vi "get_image.vi"(9 "Input\nparameters":T2={"Frame rate (ms)"=2000, "Worm Strain"="N2", "Time t"=0, "State"=enum."Image acquisition", "Acquisition time"=0.0, "Maximum # of images"=100000, "#TTL"=0, "time of third ttl "=100000, "ImSub Value"=0, "Time of last TTL"=0, "# Rows"=2, "# Columns"=2, "number of adjacentTTL"=0, "Sleep Deprivation status"="", "Sleep Detection"=FALSE, "Time of first sleep detection"=0, "# Sleep detections"=0, "Time max # adjacent TTL"=-10000, "Image t-1"=[], "Image t"=[]} {"# Columns" items=["1"=1, "2"=2, "3"=3, "4"=4]; "# Rows" items=["1"=1, "2"=2, "3"=3, "4"=4]}, 10 "?":bool) -> (1 "Output\nparameters":T2={"Frame rate (ms)"=2000, "Worm Strain"="N2", "Time t"=0, "State"=enum."Image acquisition", "Acquisition time"=0.0, "Maximum # of images"=100000, "#TTL"=0, "time of third ttl "=100000, "ImSub Value"=0, "Time of last TTL"=0, "# Rows"=2, "# Columns"=2, "number of adjacentTTL"=0, "Sleep Deprivation status"="", "Sleep Detection"=FALSE, "Time of first sleep detection"=0, "# Sleep detections"=0, "Time max # adjacent TTL"=-10000, "Image t-1"=[], "Image t"=[]} {"# Columns" items=["1"=1, "2"=2, "3"=3, "4"=4]; "# Rows" items=["1"=1, "2"=2, "3"=3, "4"=4]}, 5 "Intensity Graph":u16[][](graph))   [LabVIEW 2011]
uses:
  state.ctl
panel:
  out "?":i32
  out "?":i32
  # "General settings"
  # "Select number of animals"
  # "Row"
  # "Column"
  # "General settings"
  # "Select number of animals"
  # "Row"
  # "Column"
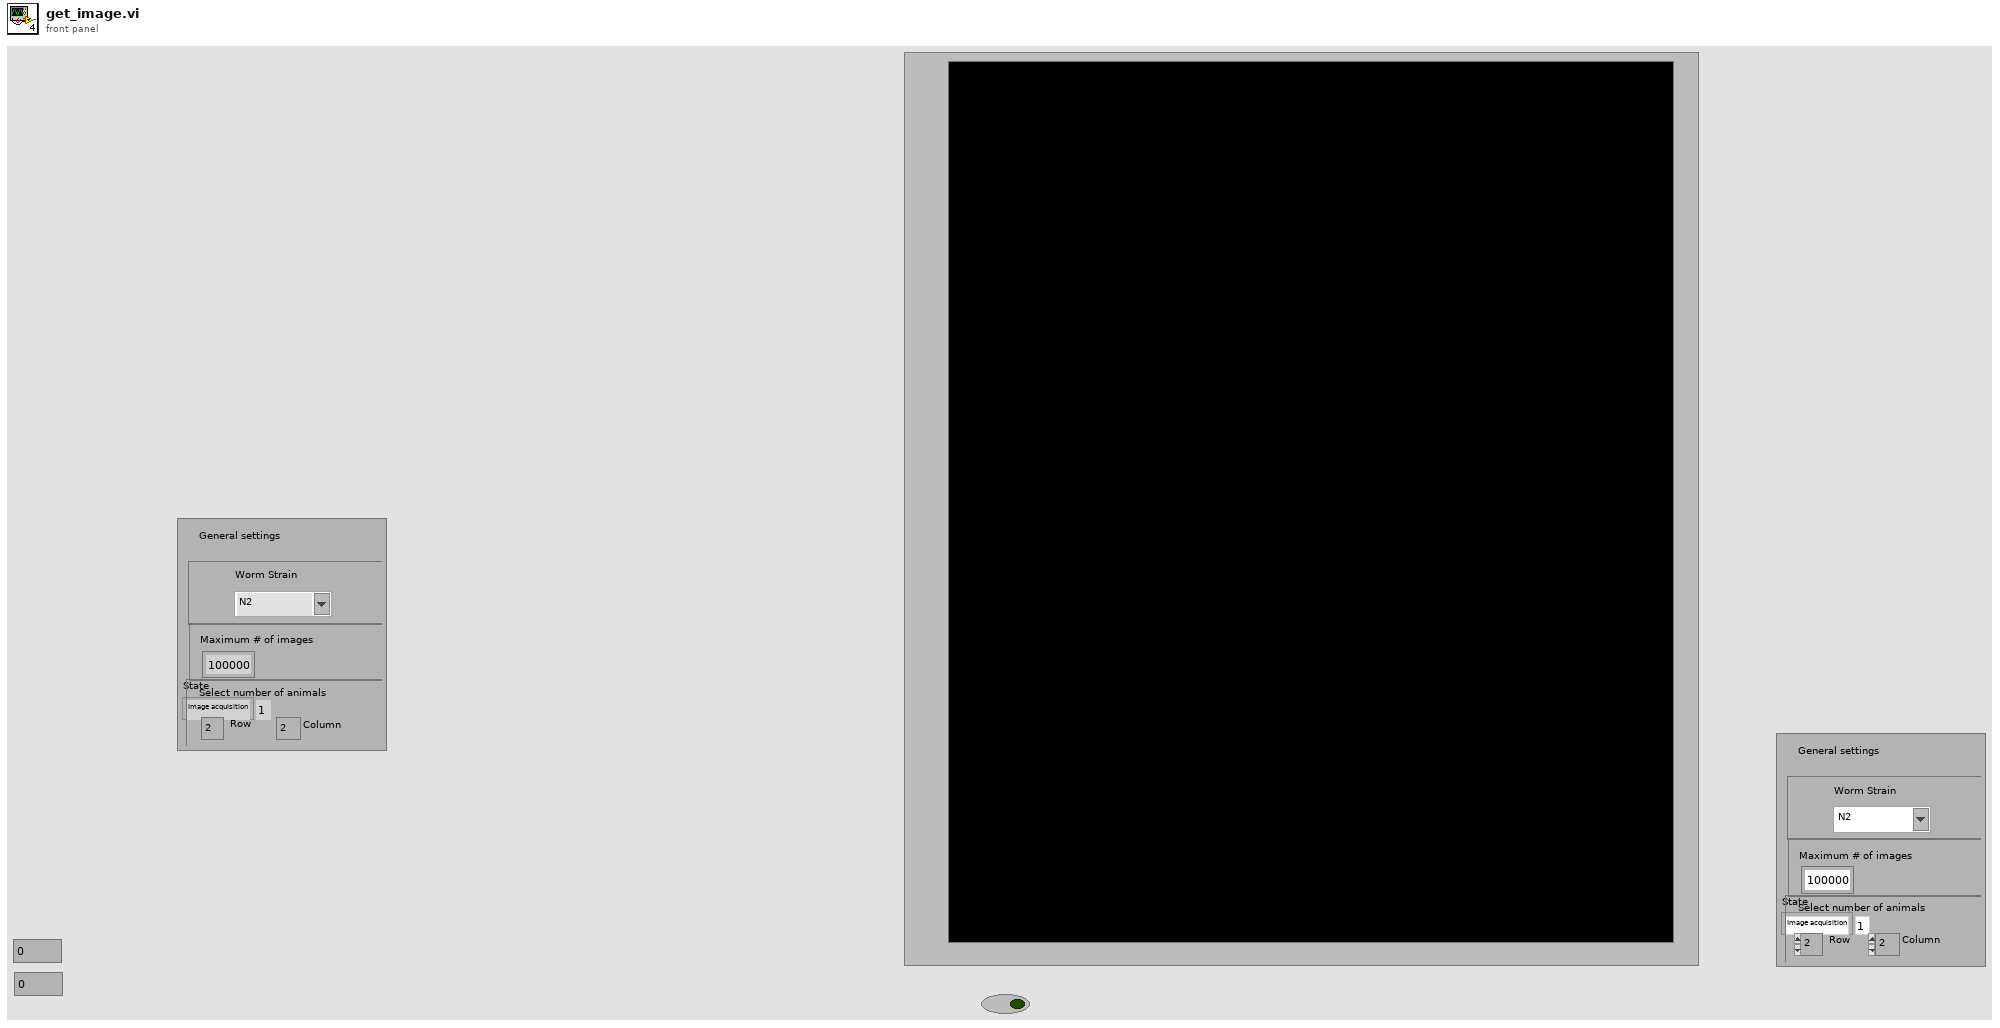
[diagram p1: front panel]
types:
  T1 = typedef "state.ctl" = enum16{"Initialize measurement", "Image acquisition", "Image processing", "Sleep detection", "Control TTL protocol ", "Sleep deprivation", "Update image & exit condition", "Wait "}
  T2 = cluster{"Frame rate (ms)":u32, "Worm Strain":string, "Time t":i32, "State":T1, "Acquisition time":dbl, "Maximum # of images":i32, "#TTL":i32, "time of third ttl ":i32, "ImSub Value":i32, "Time of last TTL":i32, "# Rows":u32, "# Columns":u32, "number of adjacentTTL":i32, "Sleep Deprivation status":string, "Sleep Detection":bool, "Time of first sleep detection":i32, "# Sleep detections":i32, "Time max # adjacent TTL":i32, "Image t-1":i32[][], "Image t":i32[][]}
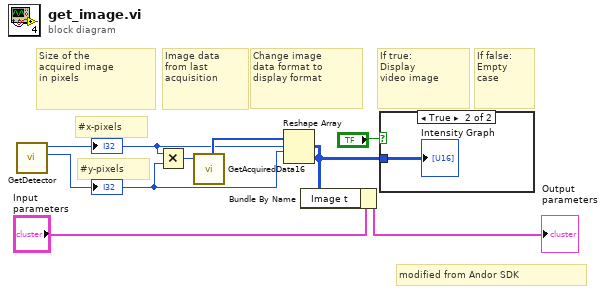
[diagram p0: block diagram]
diagram:
  # "modified from Andor SDK"
  # "Change image \ndata format to \ndisplay format"
  # "#y-pixels"
  # "#x-pixels"
  # "Image data\nfrom last\nacquisition"
  # "Size of the\nacquired image \nin pixels"
  # "If false:\nEmpty \ncase"
  # "If true: \nDisplay\nvideo image"
  n1 = call <userlib>:"GetDetector.vi"() -> ("ypixels"=w3:i32, "xpixels"=w2:i32)  [unwired: 4 in, 2 out]
  "?" <- w2
  "?" <- w3
  n2 = Multiply(x=w2, y=w3) -> (x*y=w8:i32)
  n3 = call <userlib>:"GetAcquiredData16.vi"("size"=w8) -> ("array"=w4:u16[])  [unwired: 2 in, 2 out]
  n4 = Reshape Array(w4, w3, w2) -> (w6:u16[][])
  n5 = Bundle By Name(cluster="Input\nparameters", "Image t"=w6) -> (→"Output\nparameters":T2)
  n6 = case shown="True" "?" {
    tunnel: w6 -> [_ w9]
    frame False {
    }
    frame True {
      "Intensity Graph" <- w9
    }
  }
